vi "oa_Perform Peak Average and Weighting.vi"(8 "averages completed":dbl format="%.2f", 9 "number of averages":u32=10 min=1 step=1, 10 "previous array":dbl[](array[numeric]), 11 "Y":dbl[][](array[numeric])) -> (0 "averages completed out":dbl format="%.2f", 1 "average done?":bool, 3 "power spectrum":dbl[](array[numeric]))   [LabVIEW 2017, in "SoundVib_Resampling.lvlib"]
uses:
  <vilib>/addons/Sound and Vibration/Order Analysis/Resample Order Tracking/SoundVib_Resampling.lvlib
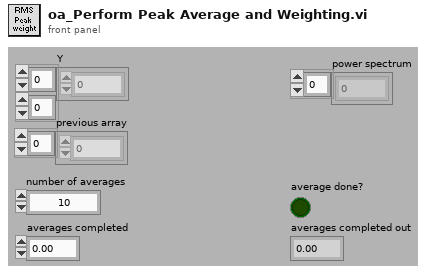
[diagram p1: front panel]
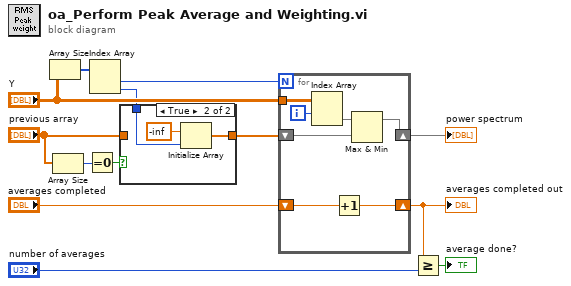
[diagram p0: block diagram]
diagram:
  n1 = Array Size(array="Y") -> (size(s)=w8:i32[])
  n2 = Array Size(array="previous array") -> (size(s)=w6:i32)
  n3 = Equal To 0?(x=w6) -> (x = 0?=w5:bool)
  n4 = Index Array(array=w8) -> (element #1=w1:i32, element #2=w2:i32)  [unwired: 2 in]
  n5 = case shown="True" w5 {
    tunnel: "previous array" -> [w14 _]
    tunnel: [w14 w15] -> w3
    tunnel: w2 -> [_ w17]
    frame False {
    }
    frame True {
      n6 = Initialize Array(-inf ("element"), w17) -> (w15:dbl[])
    }
  }
  n7 = for {
    N: w1 -> [_]
    tunnel: "Y" -> [w22]
    shift-right: [w23] -> w12
    shift-left: "averages completed" -> [w24]
    shift-right: [w18] -> w7
    shift-left: w3 -> [w19]
    i -> [w21]
    n8 = Index Array(array=w22, index (row)=w21) -> (element=w20:dbl[])  [unwired: 1 in]
    n9 = Increment(x=w24) -> (x+1=w23:dbl)
    n10 = Max & Min(x=w20, y=w19) -> (max(x,y)=w18:dbl[])  [unwired: 1 out]
  }
  "power spectrum" <- w7
  "averages completed out" <- w12
  n11 = Greater Or Equal?(x=w12, y="number of averages") -> (x >= y?=→"average done?":bool)
